vi "Modified - Artificial Strip Chart.vi"() -> (3 "Output 2D Image":picture)   [LabVIEW 2017]
doc: "Uses the Plot XY VI to create an XY strip chart in a picture indicator. Because you cannot scroll an arbitrary region of a picture, the VI maintains a limited history of points, and draws them as a graph with each update."
panel:
  in  "Stop":bool
  out "2D Picture":picture
  # "Overview: Uses the Plot XY VI to create an XY strip chart in a picture indicator. \nInstructions:\n1. Run the VI.\n2. Click Stop to stop the VI."
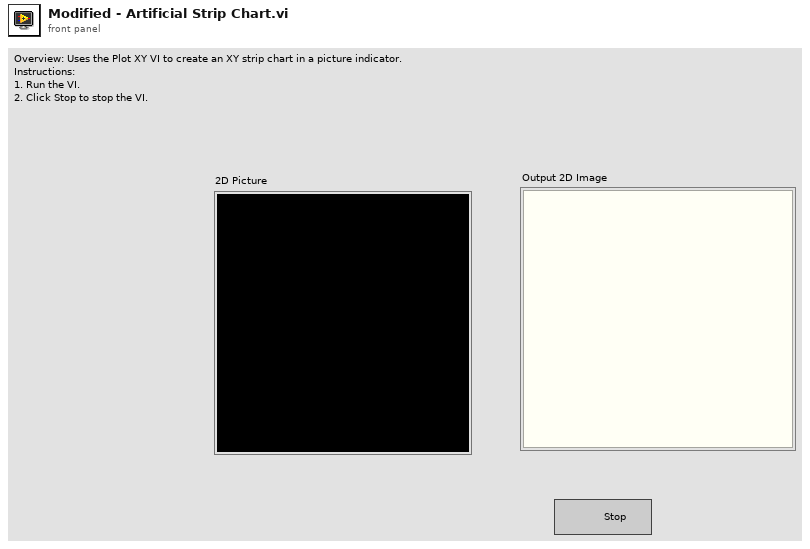
[diagram p1: front panel]
types:
  T1 = cluster{"Initial X Value":dbl, "Initial X Value":dbl}
  T2 = cluster{"Initial X Value":dbl, "Initial X Value":dbl}[]
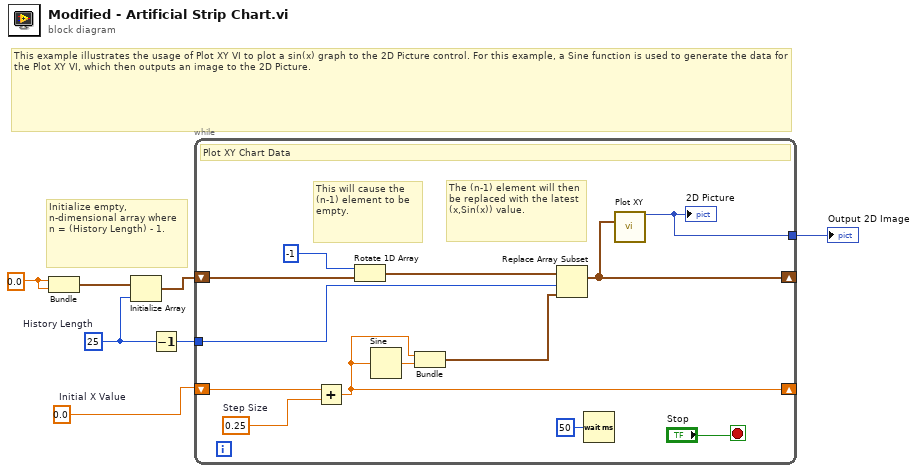
[diagram p0: block diagram]
diagram:
  w5 = 0.0 ("Initial X Value")
  w6 = 0.0  # Initial X Value
  w3 = 25  # History Length
  # "This example illustrates the usage of Plot XY VI to plot a sin(x) graph to the 2D Picture control. For this example, a Sine function is used to generate the data for the Plot XY VI, which then outputs an image to the 2D Picture."
  # "Initialize empty, n-dimensional array where n = (History Length) - 1."
  n1 = Bundle("Initial X Value"=w5, "Initial X Value"=w5) -> (w4:T1)  [unwired: 1 in]
  n2 = Initialize Array(w4, w3) -> (w2:T2)
  n3 = Decrement(x=w3) -> (x-1=w7:i32)
  n4 = while {
    shift-right: [w15] -> _
    shift-left: w2 -> [w20]
    tunnel: w7 -> [w18]
    shift-right: [w14] -> _
    shift-left: w6 -> [w16]
    tunnel: [w8] -> w1
    stop <- "Stop" stop-if-true
    w9 = 0.25  # Step Size
    # "The (n-1) element will then be replaced with the latest (x,Sin(x)) value."
    # "This will cause the (n-1) element to be empty."
    # "Plot XY Chart Data"
    n5 = Add(x=w16, y=w9) -> (x+y=w14:dbl)
    n6 = Rotate 1D Array(1:w20, 2:-1) -> (0:w10:T2)
    n7 = Sine(x=w14) -> (sin(x)=w17:dbl)
    n8 = Bundle(w14, w17) -> (w11:cluster{dbl, dbl})  [unwired: 1 in]
    n9 = Replace Array Subset(array=w10, new element=w11, index=w18) -> (w15:T2)
    n10 = Wait (ms)(milliseconds to wait=u32 50 ("millisecond multiple")) -> ()  [unwired: 1 out]
    n11 = call <vilib>:"Plot XY.vi"("data"=w15) -> ("new picture"=w8:picture)  [unwired: 14 in]
    "2D Picture" <- w8
  }
  "Output 2D Image" <- w1
